vi "Actor Core.vi"(8 "error in":errorcluster, 11 "Nested in":refnum<class "ACQ Generador.lvclass">) -> (0 "error out":errorcluster, 3 "Actor out":refnum<class "Actor.lvclass">)   [LabVIEW 2020, in "ACQ Generador.lvlib" / "ACQ Generador.lvclass"]
doc: "(<B>Filename</B>: Actor Framework.lvlib:Actor.lvclass:Actor Core.vi)\n\nReceives messages to the actor, reacts to them, and initiates any error handling that may shut the actor down.\n\nDescendant classes may override this VI to append parallel tasks for the actor to complete while it handles messages. Overrides use the Call Parent Method node."
uses:
  ACQ Generador.lvclass
  C:/Program Files (x86)/National Instruments/LabVIEW 2020/vi.lib/ActorFramework/Actor/Actor.lvclass
  <vilib>/ActorFramework/Actor/Actor.lvclass
  <vilib>/ActorFramework/Actor/Actor.lvclass/Actor.ctl
  ACQ Generador.lvclass/ACQ Generador.ctl
  Generador Messages/Graph Msg/Graph Msg.lvclass/Graph Msg.ctl
  <vilib>/ActorFramework/Message Enqueuer/Message Enqueuer.lvclass/Message Enqueuer.ctl
  <vilib>/ActorFramework/Message Enqueuer/Enqueue.vi
  Generador Messages/Graph Msg/Graph Msg.lvclass
  C:/Program Files (x86)/National Instruments/LabVIEW 2020/vi.lib/ActorFramework/Message/Message.lvclass
  <vilib>/ActorFramework/Stop Msg/Stop Msg.lvclass
  <vilib>/ActorFramework/Message Priority Queue/Priority Enqueue.vi
  <vilib>/measure/NI_MABase.lvlib
types:
  T1 = cluster{"Stop":refnum<user-event>, "Start/Stop":refnum<user-event>, "Signal":refnum<user-event>, "Amplitude":refnum<user-event>, "Frequency":refnum<user-event>}
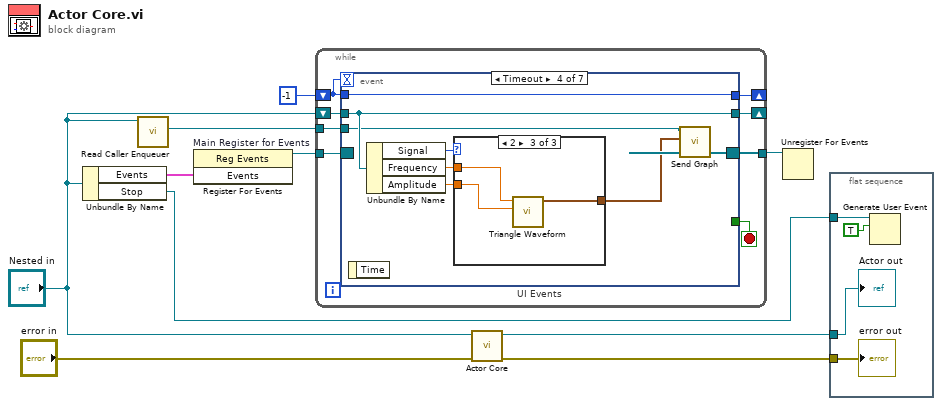
[diagram p0: block diagram]
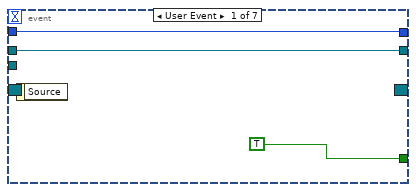
[diagram p2: hidden frame]
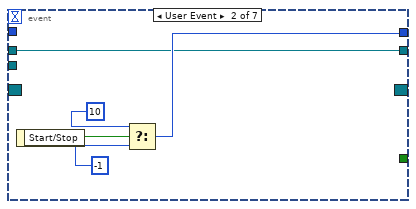
[diagram p3: hidden frame]
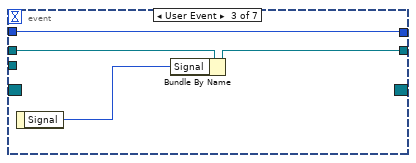
[diagram p4: hidden frame]
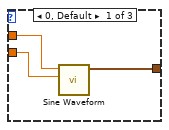
[diagram p5: hidden frame]
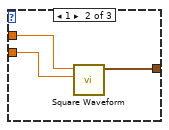
[diagram p6: hidden frame]
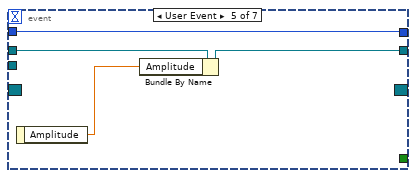
[diagram p7: hidden frame]
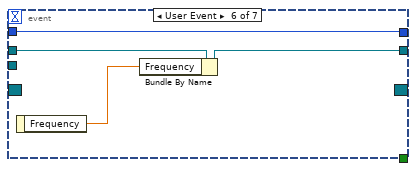
[diagram p8: hidden frame]
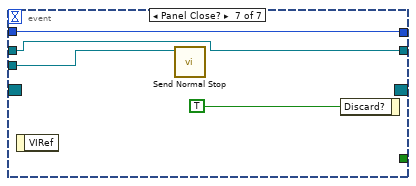
[diagram p9: hidden frame]
diagram:
  n1 = Unbundle By Name("Nested in") -> ("Events"=w7:T1, "Stop"=w4:refnum<user-event>)
  n2 = call <vilib>:"Read Caller Enqueuer.vi"("Actor"="Nested in") -> ("Caller Enqueuer"=w1:refnum<class "Message Enqueuer.lvclass">)  [unwired: 10 in]
  n3 = register-events "Main Register for Events"(w7) -> (reference out=w8:refnum<event-registration>)  [unwired: 2 in, 1 out]
  n4 = while {
    tunnel: w8 -> [w18]
    tunnel: [w16] -> w6
    tunnel: w1 -> [w15]
    shift-right: [w14] -> _
    shift-left: -1 -> [w13]
    shift-right: [w11] -> _
    shift-left: "Nested in" -> [w12]
    stop <- w17 stop-if-true
    n5 = event "UI Events" shown="[3] Timeout" {
      selector: w18 -> [_ _ _ _ _ _ _]
      dyn-events: [_ _ _ _ _ _ _] -> w16
      timeout: w13 -> [_ _ _ _ _ _ _]
      tunnel: [TRUE _ _ _ _ _ _] -> w17
      tunnel: w15 -> [_ _ _ w32 _ _ w57]
      tunnel: [w20 w23 w30 w37 w50 w54 w56] -> w14
      tunnel: w13 -> [w20 _ w30 w37 w50 w54 w56]
      tunnel: w12 -> [w19 w22 w29 w33 w49 w53 w55]
      tunnel: [w19 w22 w28 w33 w48 w52 w55] -> w11
      event User Event {
        n6 = event-data() -> ()  [unwired: 1 in, 1 out]
      }
      event User Event {
        n7 = event-data() -> ("Start/Stop"=w26:bool)  [unwired: 1 in]
        n8 = Select(t=10, s=w26, f=-1) -> (s? t:f=w23:i32)
      }
      event User Event {
        n9 = event-data() -> ("Signal"=w27:u16)  [unwired: 1 in]
        n10 = Bundle By Name(cluster=w29, "Signal"=w27) -> (w28:refnum<class "ACQ Generador.lvclass">)
      }
      event Timeout {
        n11 = event-data() -> ()  [unwired: 1 in, 1 out]
        n12 = Unbundle By Name(w33) -> ("Signal"=w36:u16, "Frequency"=w35:dbl, "Amplitude"=w34:dbl)
        n13 = case shown="2" w36 {
          tunnel: w35 -> [w40 w43 w46]
          tunnel: w34 -> [w39 w42 w45]
          tunnel: [w38 w41 w44] -> w31
          frame 0, Default {
            n14 = call <vilib>:"Sine Waveform.vi"("amplitude"=w39, "frequency"=w40) -> ("signal out"=w38:waveform(dbl))  [unwired: 8 in, 1 out]
          }
          frame 1 {
            n15 = call <vilib>:"Square Waveform.vi"("amplitude"=w42, "frequency"=w43) -> ("signal out"=w41:waveform(dbl))  [unwired: 8 in, 1 out]
          }
          frame 2 {
            n16 = call <vilib>:"Triangle Waveform.vi"("amplitude"=w45, "frequency"=w46) -> ("signal out"=w44:waveform(dbl))  [unwired: 8 in, 1 out]
          }
        }
        n17 = call "Send Graph.vi"("signal out"=w31, "Message Enqueuer"=w32) -> ()  [unwired: 8 in, 2 out]
      }
      event User Event {
        n18 = event-data() -> ("Amplitude"=w47:dbl)  [unwired: 1 in]
        n19 = Bundle By Name(cluster=w49, "Amplitude"=w47) -> (w48:refnum<class "ACQ Generador.lvclass">)
      }
      event User Event {
        n20 = event-data() -> ("Frequency"=w51:dbl)  [unwired: 1 in]
        n21 = Bundle By Name(cluster=w53, "Frequency"=w51) -> (w52:refnum<class "ACQ Generador.lvclass">)
      }
      event Panel Close? {
        n22 = event-data() -> ()  [unwired: 1 in, 1 out]
        n23 = call <vilib>:"Send Normal Stop.vi"("Message Enqueuer"=w57) -> ()  [unwired: 10 in, 1 out]
        n24 = event-data("Discard?"=TRUE) -> ()  [unwired: 1 in, 1 out]
      }
    }
  }
  n25 = call-parent "Actor Core.vi"("error in"="error in", "Actor in"="Nested in") -> ("error out"=w10:errorcluster, "Actor out"=w9:refnum<class "Actor.lvclass">)  [unwired: 8 in]
  n26 = Unregister For Events(event registration refnum=w6) -> ()  [unwired: 1 in, 1 out]
  n27 = flat-sequence {
    tunnel: w10 -> [w62]
    tunnel: w9 -> [w61]
    tunnel: w4 -> [w60]
    frame #0 {
      n28 = Generate User Event(user event=w60, event data cluster=TRUE ("event data")) -> ()  [unwired: 2 in, 2 out]
      "error out" <- w62
      "Actor out" <- w61
    }
  }
